vi "PiezoSignal.vi"(0 "Piezo Position (um)":dbl, 1 "Exposure (ms)":dbl=10.0 format="%0.2p", 2 "Samples /Millisecond":dbl=10.0 format="%0.2p", 3 "Relax (ms)":dbl=10.0 format="%0.2p", 4 "Underscan /ms":dbl, 5 "Camera Delay /ms":dbl) -> (7 "Signal":dbl[](array[numeric]))   [LabVIEW 2015]
panel:
  out "Piezo Signal 2":dbl[](graph)
  out "Piezo Signal":dbl[](graph)
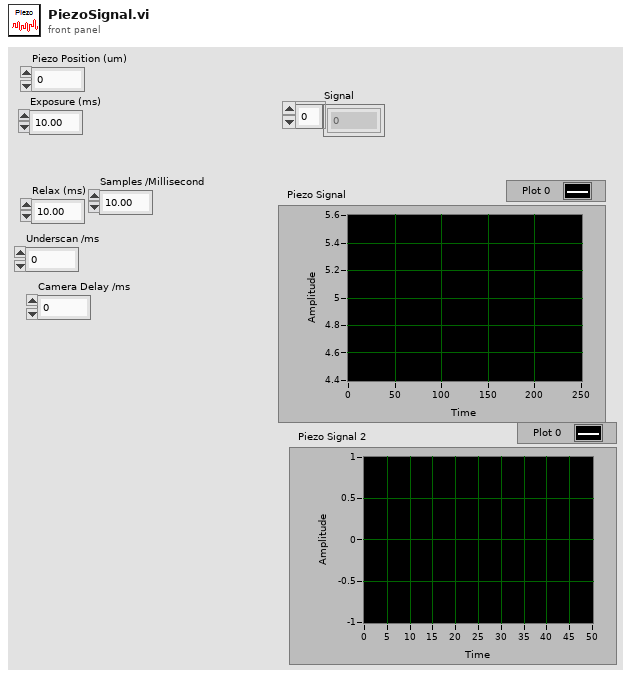
[diagram p1: front panel]
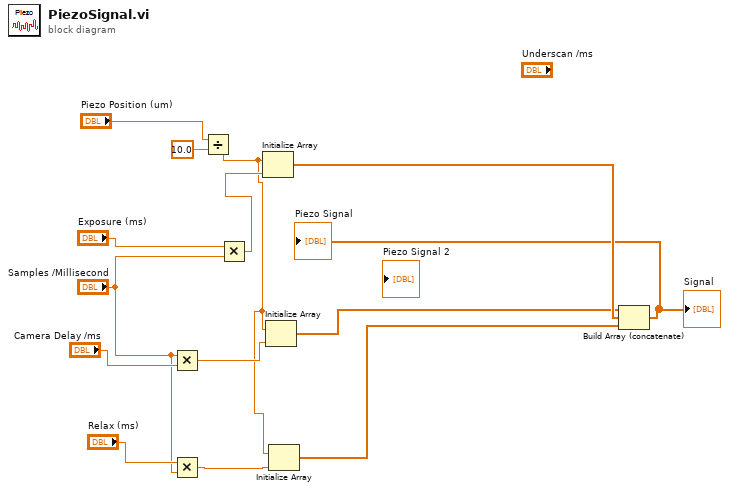
[diagram p0: block diagram]
diagram:
  n1 = Multiply(x="Samples /Millisecond", y="Camera Delay /ms") -> (x*y=w2:dbl)
  n2 = Multiply(x="Relax (ms)", y="Samples /Millisecond") -> (x*y=w7:dbl)
  n3 = Divide(x="Piezo Position (um)", y=10.0) -> (x/y=w1:dbl)
  n4 = Multiply(x="Exposure (ms)", y="Samples /Millisecond") -> (x*y=w11:dbl)
  n5 = Initialize Array(w1, w11) -> (w6:dbl[])
  n6 = Initialize Array(w1, w2) -> (w4:dbl[])
  n7 = Initialize Array(w1, w7) -> (w3:dbl[])
  n8 = Build Array (concatenate)(w4, w6, w3) -> (→"Signal" →"Piezo Signal":dbl[])
